vi "NI-test-write.vi"() -> ()   [LabVIEW 2014]
uses:
  <vilib>/Utility/error.llb/DialogType.ctl
  <vilib>/DAQmx/create/channels.llb/DAQmx Create Channel (AO-Voltage-Basic).vi
  <vilib>/DAQmx/configure/timing.llb/DAQmx Timing (Sample Clock).vi
  <vilib>/DAQmx/configure/trigger.llb/DAQmx Start Trigger (Digital Edge).vi
  <vilib>/DAQmx/configure/trigger.llb/DAQmx Start Trigger (Analog Edge).vi
  <vilib>/DAQmx/write.llb/DAQmx Write (Analog 1D Wfm NChan NSamp).vi
  <resource>/objmgr/daqmx.rc
  <vilib>/measure/NI_MABase.lvlib
panel:
  out "Waveform Graph":waveform(dbl)[](graph)=[{"t0"=timestamp(0 s since 1904-01-01), "dt"=0.001, "Y"=[]}]
  in  "Output Array":T1(array[cluster])=[{"Waveform Type"=0, "Amplitude"=1.0, "Frequency"=10.0}] {"Frequency" format="%0.2p"; "Amplitude" format="%0.2p"; "Waveform Type" items=["Sine Wave", "Triangle Wave", "Square Wave", "Sawtooth Wave"]}
  in  "Number of Samples":i32=1000
  in  "Trigger Type":T2(tab)
  in  "Edge":i32(ring)=10280 items=["Rising"=10280, "Falling"=10171]
  in  "Digital Trigger Source":tag
  in  "Level (V)":dbl format="%0.2f"
  in  "Hysteresis (V)":dbl
  in  "Slope":i32(ring)=10280 items=["Rising"=10280, "Falling"=10171]
  in  "Analog Trigger Source":string="APFI0"
  in  "Pause When":i32(ring)=10192 items=["High"=10192, "Low"=10214]
  in  "Pause Trigger Source":tag
  in  "Sample Rate":dbl=1000.0
  in  "Sample Clock Source":tag="OnboardClock"
  in  "Max Voltage":dbl=5.0
  in  "Min Voltage":dbl=-5.0
  in  "Physical Channel(s)":tag="Dev1/ao0"
  out "Actual Sample Rate":dbl=1000.0 format="%0.2f"
  in  "Stop":bool
  # "To configure and use a start trigger you must have the necessary tab selected above.  Not all hardware supports triggering--refer to your device documentation for more info."
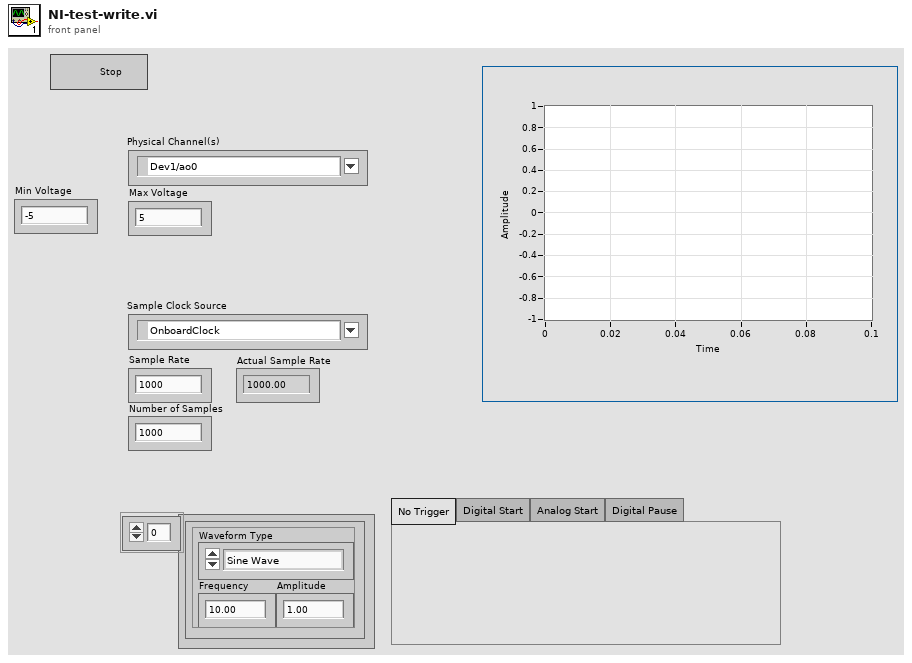
[diagram p1: front panel]
types:
  T1 = cluster{"Waveform Type":u16, "Amplitude":dbl, "Frequency":dbl}[]
  T2 = enum32{"No Trigger", "Digital Start", "Analog Start", "Digital Pause"}
  T3 = typedef "DialogType.ctl" = u16
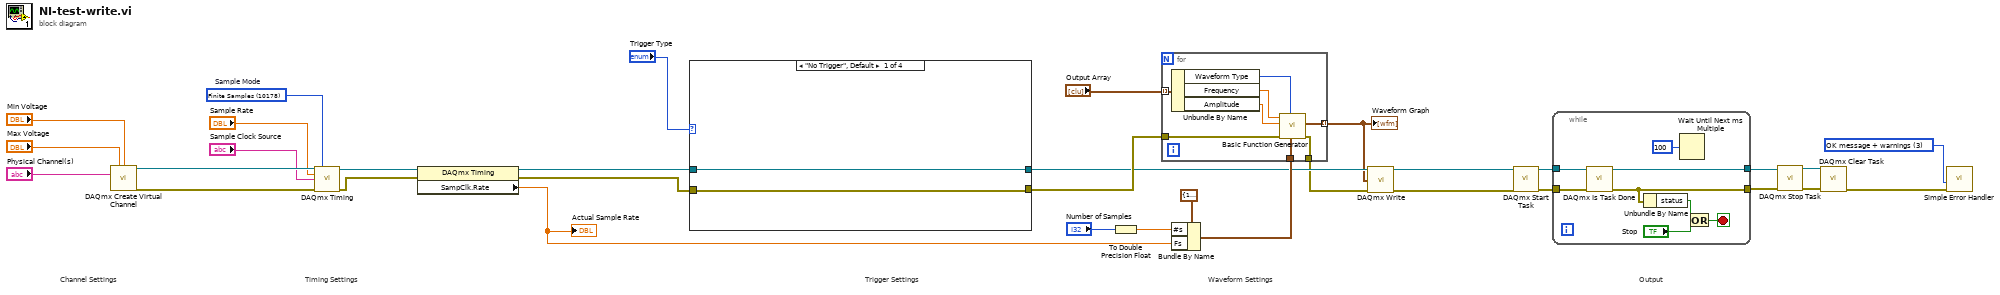
[diagram p0: block diagram]
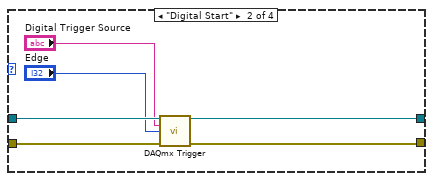
[diagram p2: hidden frame]
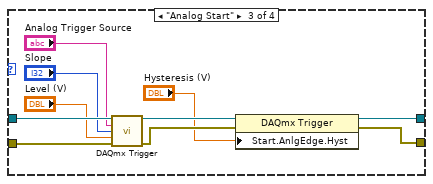
[diagram p3: hidden frame]
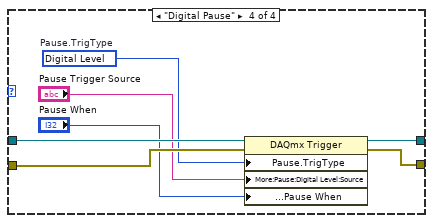
[diagram p4: hidden frame]
diagram:
  w1 = T3 3 items=["no dialog", "OK message", "continue or stop message", "OK message + warnings", "continue/stop + warnings"] ("type of dialog (OK msg:1)")
  w31 = 10178 items=["Finite Samples"=10178, "Continuous Samples"=10123, "Hardware Timed Single Point"=12522]  # Sample Mode
  # "Output"
  # "Trigger Settings"
  # "Waveform Settings"
  # "Timing Settings"
  # "Channel Settings"
  n1 = call-poly <vilib>:"DAQmx Create Virtual Channel.vi"("maximum value"="Max Voltage", "minimum value"="Min Voltage", "physical channels"="Physical Channel(s)") -> ("task out"=w29:refnum<k21>, "error out"=w30:errorcluster)  [unwired: 11 in]
  n2 = call-poly <vilib>:"DAQmx Timing.vi"("task/channels in"=w29, "sample mode"=w31, "rate"="Sample Rate", "source"="Sample Clock Source", "error in"=w30) -> ("task out"=w33:refnum<k21>, "error out"=w32:errorcluster)  [unwired: 9 in]
  n3 = property class="DAQmx Timing"(reference=w33, error in=w32) -> (reference out=w19:refnum<k21>, error out=w18:errorcluster, "SampClk.Rate"=w15:dbl)
  "Actual Sample Rate" <- w15
  n4 = case shown="\"No Trigger\", Default" "Trigger Type" {
    tunnel: w19 -> [w35 w41 w51 w58]
    tunnel: w18 -> [w34 w40 w50 w55]
    tunnel: [w35 w39 w48 w57] -> w13
    tunnel: [w34 w38 w47 w56] -> w17
    frame "No Trigger", Default {
    }
    frame "Digital Start" {
      n5 = call-poly <vilib>:"DAQmx Trigger.vi"("task/channels in"=w41, "source"="Digital Trigger Source", "edge"="Edge", "error in"=w40) -> ("task out"=w39:refnum<k21>, "error out"=w38:errorcluster)  [unwired: 10 in]
    }
    frame "Analog Start" {
      n6 = call-poly <vilib>:"DAQmx Trigger.vi"("task/channels in"=w51, "source"="Analog Trigger Source", "slope"="Slope", "level"="Level (V)", "error in"=w50) -> ("task out"=w46:refnum<k21>, "error out"=w45:errorcluster)  [unwired: 9 in]
      n7 = property class="DAQmx Trigger"(reference=w46, error in=w45, "Start.AnlgEdge.Hyst"="Hysteresis (V)") -> (reference out=w48:refnum<k21>, error out=w47:errorcluster)
    }
    frame "Digital Pause" {
      w54 = 10152 items=["Analog Level"=10101, "Analog Window"=10103, "Digital Level"=10152, "Digital Pattern"=10398, "None"=10230]  # Pause.TrigType
      n8 = property class="DAQmx Trigger"(reference=w58, error in=w55, "Pause.TrigType"=w54, "More:Pause:Digital Level:Source"="Pause Trigger Source", "More:Pause:Digital Level:Pause When"="Pause When") -> (reference out=w57:refnum<k21>, error out=w56:errorcluster)
    }
  }
  n9 = To Double Precision Float(number="Number of Samples") -> (double precision float=w7:dbl)
  n10 = Bundle By Name(cluster=cluster{"Fs":dbl, "#s":dbl} {"Fs"=1000.0, "#s"=1000.0} ("sampling info"), "#s"=w7, "Fs"=w15) -> (w14:cluster{"Fs":dbl, "#s":dbl})
  n11 = for {
    tunnel: w17 -> [w66]
    tunnel: w14 -> [w65]
    tunnel: [w64] -> w10
    tunnel: "Output Array" -> [w63] mode=indexing
    tunnel: [w59] -> w8 mode=indexing
    n12 = Unbundle By Name(w63) -> ("Waveform Type"=w62:u16, "Frequency"=w61:dbl, "Amplitude"=w60:dbl)
    n13 = call <vilib>:"Basic Function Generator.vi"("sampling info"=w65, "signal type"=w62, "error in (no error)"=w66, "amplitude"=w60, "frequency"=w61) -> ("error out"=w64:errorcluster, "signal out"=w59:waveform(dbl))  [unwired: 4 in, 1 out]
  }
  "Waveform Graph" <- w8
  n14 = call-poly <vilib>:"DAQmx Write.vi"("task/channels in"=w13, "data"=w8, "error in"=w10) -> ("task out"=w12:refnum<k21>, "error out"=w11:errorcluster)  [unwired: 10 in, 1 out]
  n15 = call <vilib>:"DAQmx Start Task.vi"("task/channels in"=w12, "error in"=w11) -> ("task out"=w28:refnum<k21>, "error out"=w27:errorcluster)  [unwired: 12 in]
  n16 = while {
    tunnel: w28 -> [w74]
    tunnel: w27 -> [w73]
    tunnel: [w70] -> w2
    tunnel: [w71] -> w3
    stop <- w72 stop-if-true
    n17 = call <vilib>:"DAQmx Is Task Done.vi"("task/channels in"=w74, "error in"=w73) -> ("task out"=w71:refnum<k21>, "error out"=w70:errorcluster)  [unwired: 11 in, 1 out]
    n18 = Unbundle By Name(w70) -> ("status"=w69:bool)
    n19 = Wait Until Next ms Multiple(millisecond multiple=u32 100) -> ()  [unwired: 1 out]
    n20 = Or(x=w69, y="Stop") -> (x .or. y?=w72:bool)
  }
  n21 = call <vilib>:"DAQmx Stop Task.vi"("task/channels in"=w3, "error in"=w2) -> ("task out"=w5:refnum<k21>, "error out"=w4:errorcluster)  [unwired: 12 in]
  n22 = call <vilib>:"DAQmx Clear Task.vi"("task in"=w5, "error in"=w4) -> ("error out"=w26:errorcluster)  [unwired: 13 in]
  n23 = call <vilib>:"Simple Error Handler.vi"("type of dialog (OK msg:1)"=w1, "error in (no error)"=w26) -> ()  [unwired: 3 in, 5 out]
